vi "Array of clusters.vi"() -> ()   [LabVIEW 2021]
uses:
  <vilib>/measure/NI_MAPro.lvlib
  <vilib>/measure/maspectr.llb/FFT Spectrum (Real-Im) for 1 Chan.vi
  <vilib>/Analysis/4window.llb/windowTd.ctl
  <vilib>/Analysis/NI_AALPro.lvlib
panel:
  out "element":cluster{"f0":dbl, "df":dbl, "real part":dbl[]}
  in  "window 2":T1=1 items=["Rectangle"=0, "Hanning"=1, "Hamming"=2, "Blackman-Harris"=3, "Exact Blackman"=4, "Blackman"=5, "Flat Top"=6, "4 Term B-Harris "=7, "7 Term B-Harris"=8, "Low Sidelobe"=9, "Blackman Nuttall"=11, "Triangle"=30, "Bartlett-Hanning"=31, "Bohman"=32, "Parzen"=33, "Welch"=34, "Kaiser"=60, "Dolph-Chebyshev"=61, "Gaussian"=62]
  in  "window":T1=1 items=["Rectangle"=0, "Hanning"=1, "Hamming"=2, "Blackman-Harris"=3, "Exact Blackman"=4, "Blackman"=5, "Flat Top"=6, "4 Term B-Harris "=7, "7 Term B-Harris"=8, "Low Sidelobe"=9, "Blackman Nuttall"=11, "Triangle"=30, "Bartlett-Hanning"=31, "Bohman"=32, "Parzen"=33, "Welch"=34, "Kaiser"=60, "Dolph-Chebyshev"=61, "Gaussian"=62]
  out "Waveform Graph 2":dynamicdata(graph)
  out "FFT2":dynamicdata(graph)
  out "FFT1":dynamicdata(graph)
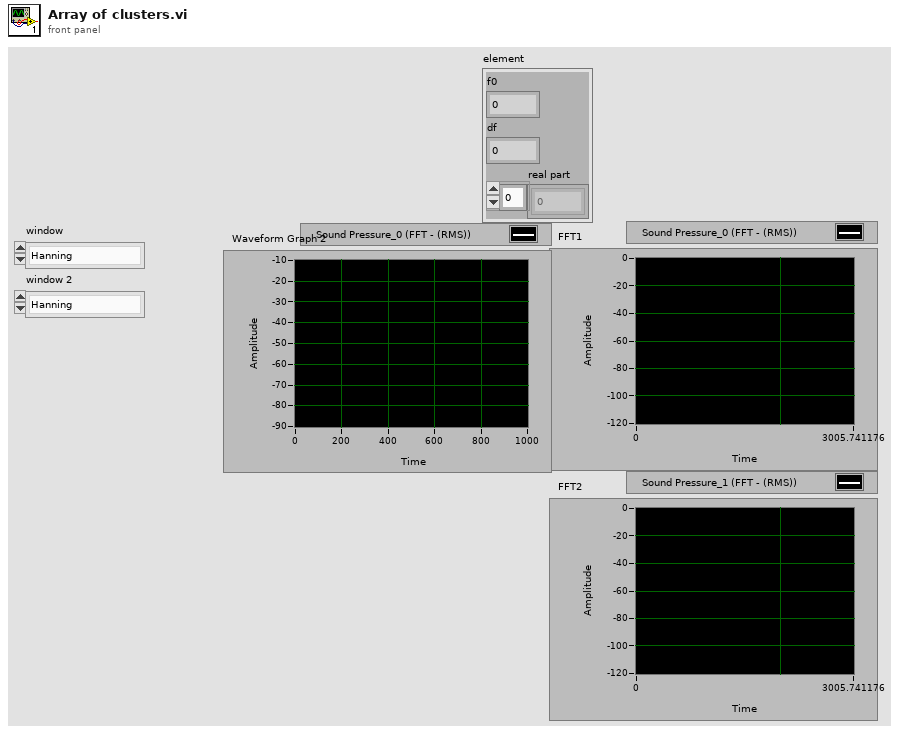
[diagram p1: front panel]
types:
  T1 = typedef "NI_AALPro.lvlib/windowTd.ctl" = u32
  T2 = cluster{"f0":dbl, "df":dbl, "imaginary part":dbl[]}
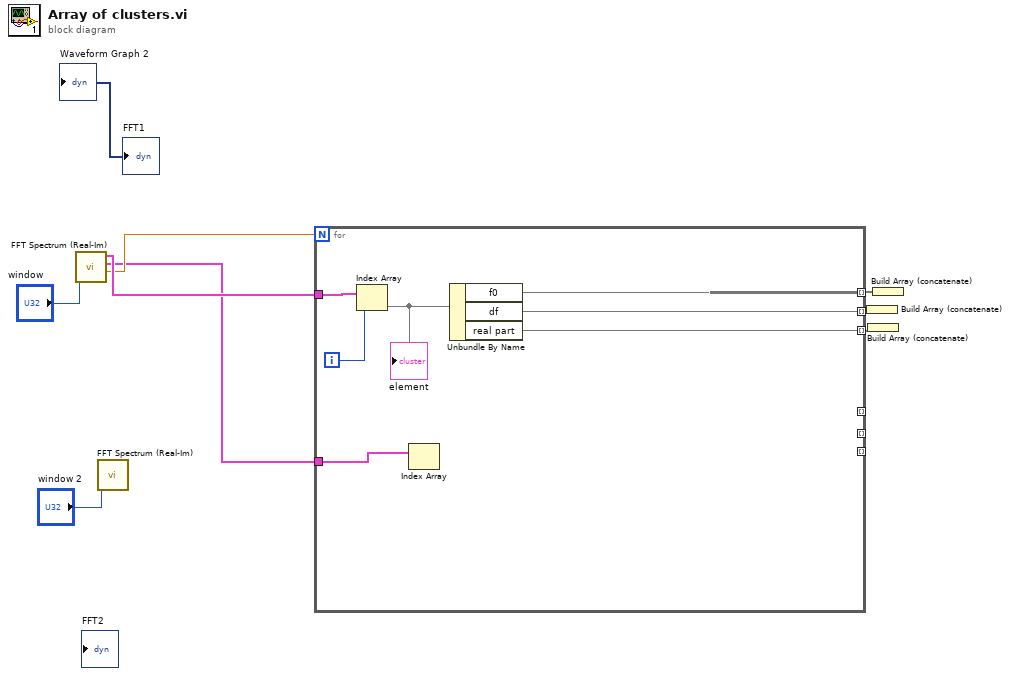
[diagram p0: block diagram]
diagram:
  n1 = call-poly <vilib>:"FFT Spectrum (Real-Im).vi"("window"="window") -> ("averages completed"=w2:dbl, "imaginary part"=w1:T2, "real part"=w6:cluster{"f0":dbl, "df":dbl, "real part":dbl[]})  [unwired: 6 in, 2 out]
  n2 = call-poly <vilib>:"FFT Spectrum (Real-Im).vi"("window"="window 2") -> ()  [unwired: 6 in, 5 out]
  n3 = for {
    N: w2 -> [_]
    tunnel: w6 -> [w12]
    tunnel: [w19] -> w5 mode=indexing
    tunnel: [w18] -> w4 mode=indexing
    tunnel: [w17] -> w3 mode=indexing
    tunnel: _ -> [w16] mode=indexing
    tunnel: _ -> [w15] mode=indexing
    tunnel: _ -> [w14] mode=indexing
    tunnel: w1 -> [w11]
    i -> [w13]
    n4 = Index Array(array=w12, index=w13) -> (element=w20)
    "element" <- w20
    n5 = Index Array(array=w11) -> ()  [unwired: 1 in, 1 out]
    n6 = Unbundle By Name(w20) -> ("f0"=w19, "df"=w18, "real part"=w17)
  }
  n7 = Build Array (concatenate)(w4) -> ()  [unwired: 1 out]
  n8 = Build Array (concatenate)(w3) -> ()  [unwired: 1 out]
  n9 = Build Array (concatenate)(w5) -> ()  [unwired: 1 out]
  "FFT1" <- "Waveform Graph 2"
